vi "RemoveNode.vi"(8 "error in":errorcluster, 10 "node":T1) -> (0 "error out":errorcluster, 2 "node ID":string)   [LabVIEW 2013, in "NISE_CEF_TreeControl.lvlib"]
doc: "Removes the node , deleting all the references to it and destroying the references"
uses:
  NISE_CEF_TreeControl.lvlib
  Node/NodeRef.ctl
  Node/NISE_CEF_Node.lvclass
  Node/NISE_CEF_Node.lvclass/NISE_CEF_Node.ctl
  Node/ReadParent.vi
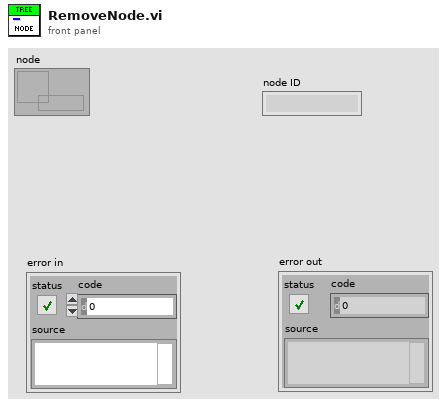
[diagram p1: front panel]
types:
  T1 = typedef "NISE_CEF_Node.lvclass/NodeRef.ctl" = refnum<data-value>
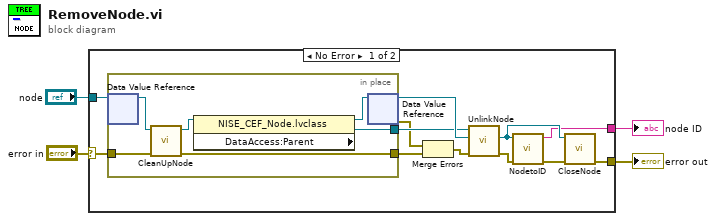
[diagram p0: block diagram]
diagram:
  n1 = case shown="No Error" "error in" {
    selector: "error in" -> [w8 w23]
    tunnel: [w10 w23] -> w3
    tunnel: "node" -> [w16 _]
    tunnel: [w9 _] -> w1
    frame No Error {
      n2 = in-place {
        in-place-border: [w21] -> w14
        in-place-border: w8 -> [w18]
        in-place-border: [w17] -> w7
        n3 = in-place-dvr #1(w16) -> (w20:refnum<class "NISE_CEF_Node.lvclass">)  [unwired: 1 out]
        n4 = call-dynamic "CleanUpNode.vi"("error in (no error)"=w18, "NISE_CEF_Node in"=w20) -> ("error out"=w17:errorcluster, "NISE_CEF_Node out"=w19:refnum<class "NISE_CEF_Node.lvclass">)  [unwired: 8 in]
        n5 = property class="NISE_CEF_Node.lvclass"(reference=w19) -> (reference out=w22:refnum<class "NISE_CEF_Node.lvclass">, "DataAccess:Parent"=w21:T1)  [unwired: 1 in, 1 out]
        n6 = in-place-dvr #1(w22) -> (w15:T1, w6:errorcluster)
      }
      n7 = Merge Errors(w6, w7) -> (w5:errorcluster)
      n8 = call "UnlinkNode.vi"("error in"=w5, "child in"=w15, "parent in"=w14) -> ("error out"=w11:errorcluster, "child out"=w12:T1)  [unwired: 6 in, 1 out]
      n9 = call "NodetoID.vi"("error in"=w11, "node ref"=w12) -> ("error out"=w13:errorcluster, "ID"=w9:string)  [unwired: 8 in]
      n10 = call "CloseNode.vi"("error in"=w13, "node ref"=w12) -> ("error out"=w10:errorcluster)  [unwired: 9 in]
    }
    frame Error {
    }
  }
  "error out" <- w3
  "node ID" <- w1
